vi "Get Ref.vi"(8 "error in (no error)":errorcluster, 11 "BetterListboxHandle in":refnum<class "BetterListboxHandle.lvclass">) -> (0 "error out":errorcluster, 2 "Tree/LB/MCL ref":refnum<vi>, 3 "BetterListboxHandle out":refnum<class "BetterListboxHandle.lvclass">)   [LabVIEW 2020, in "BetterDragAndDrop.lvlib" / "BetterListboxHandle.lvclass"]
uses:
  BetterListboxHandle.lvclass
  BetterListboxHandle.lvclass/BetterListboxHandle.ctl
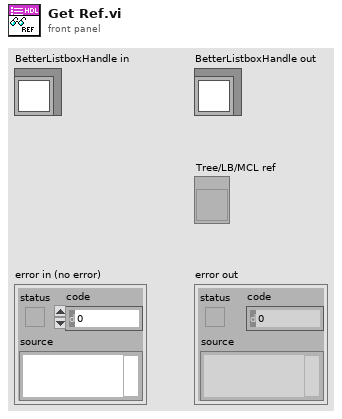
[diagram p1: front panel]
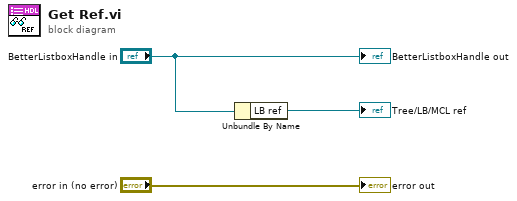
[diagram p0: block diagram]
diagram:
  n1 = Unbundle By Name("BetterListboxHandle in") -> ("LB ref"=→"Tree/LB/MCL ref":refnum<vi>)
  "error out" <- "error in (no error)"
  "BetterListboxHandle out" <- "BetterListboxHandle in"
